vi "re-register.vi"(2 "error in":errorcluster, 3 "queue":refnum<queue>) -> (0 "error out":errorcluster)   [LabVIEW 2010]
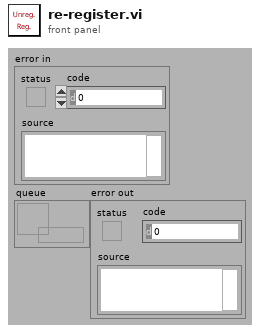
[diagram p1: front panel]
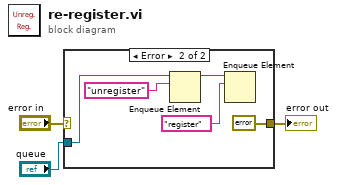
[diagram p0: block diagram]
diagram:
  n1 = case shown="Error" "error in" {
    selector: "error in" -> [w4 _]
    tunnel: "queue" -> [_ w9]
    tunnel: [w4 errorcluster {"status"=FALSE, "code"=0, "source"=""} ("error out")] -> w1
    frame No Error {
    }
    frame Error {
      n2 = Enqueue Element(queue=w9, element="unregister") -> (queue out=w8:refnum<queue>)  [unwired: 2 in, 2 out]
      n3 = Enqueue Element(queue=w8, element="register") -> ()  [unwired: 2 in, 3 out]
    }
  }
  "error out" <- w1
